vi "unregister child queue.vi"(8 "error in":errorcluster, 10 "queue":refnum<class "identifying queue.lvclass">, 11 "communicator in":refnum<class "communicator.lvclass">) -> (0 "error out":errorcluster, 3 "communicator out":refnum<class "communicator.lvclass">)   [LabVIEW 2015, in "communicator.lvclass"]
uses:
  communicator.lvclass
  communicator queue/identifying queue.lvclass
  communicator.lvclass/communicator.ctl
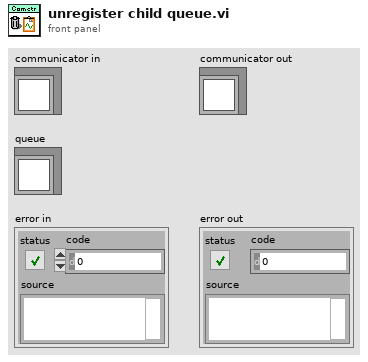
[diagram p1: front panel]
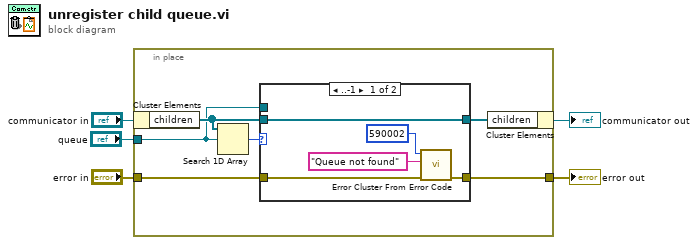
[diagram p0: block diagram]
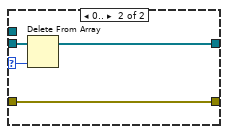
[diagram p2: hidden frame]
diagram:
  n1 = in-place {
    in-place-border: [w9] -> w3
    in-place-border: "error in" -> [w10]
    in-place-border: "queue" -> [w6]
    n2 = in-place-cluster #1("communicator in") -> ("children"=w7:refnum<class "identifying queue.lvclass">[])
    n3 = Search 1D Array(1D array=w7, element=w6) -> (index of element=w11:i32)  [unwired: 1 in]
    n4 = case shown="..-1" w11 {
      selector: w11 -> [_ w17]
      tunnel: w10 -> [w14 w20]
      tunnel: [w13 w20] -> w9
      tunnel: [w12 w18] -> w8
      tunnel: w7 -> [w12 w19]
      tunnel: w6 -> [_ _]
      frame ..-1 {
        n5 = call <vilib>:"Error Cluster From Error Code.vi"("error in (no error)"=w14, "error message (\"\")"="Queue not found" ("error message (\"\")"), "error code (0)"=590002) -> ("error out"=w13:errorcluster)  [unwired: 6 in]
      }
      frame 0.. {
        n6 = Delete From Array(array=w19, index=w17) -> (array with subset deleted=w18:refnum<class "identifying queue.lvclass">[])  [unwired: 1 in, 1 out]
      }
    }
    n7 = in-place-cluster #1("children"=w8) -> (→"communicator out":refnum<class "communicator.lvclass">)
  }
  "error out" <- w3
